vi "Read VI Refnum.vi"(8 "error in (no error)":errorcluster, 11 "Bioreactor in":refnum<class "Bioreactor.lvclass">) -> (0 "error out":errorcluster, 2 "VI Refnum":refnum<vi>, 3 "Bioreactor out":refnum<class "Bioreactor.lvclass">)   [LabVIEW 2012, in "Bioreactor Actor.lvlib" / "Bioreactor.lvclass"]
uses:
  Bioreactor.lvclass
  Bioreactor.lvclass/Bioreactor.ctl
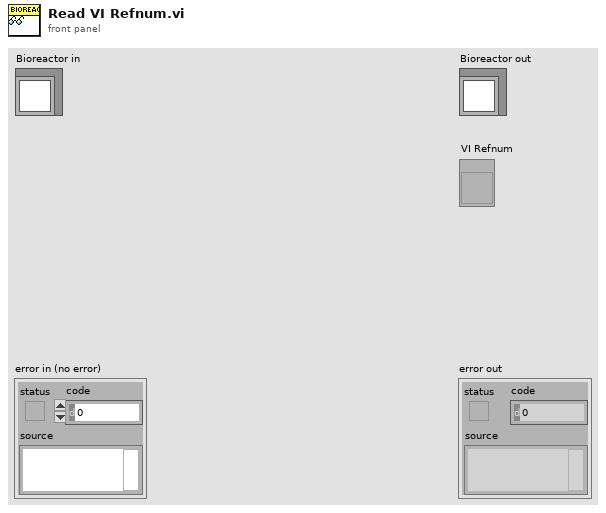
[diagram p1: front panel]
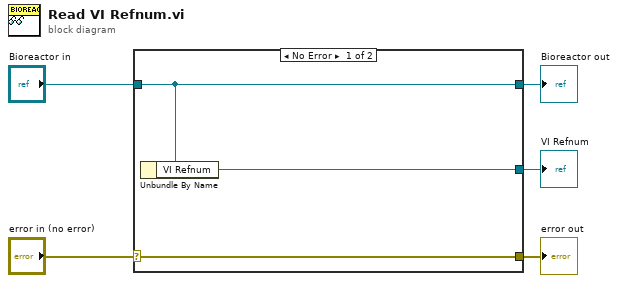
[diagram p0: block diagram]
diagram:
  n1 = case shown="No Error" "error in (no error)" {
    selector: "error in (no error)" -> [w8 w9]
    tunnel: [w8 w9] -> w4
    tunnel: [w7 w10] -> w2
    tunnel: "Bioreactor in" -> [w7 w10]
    tunnel: [w6 _] -> w1
    frame No Error {
      n2 = Unbundle By Name(w7) -> ("VI Refnum"=w6:refnum<vi>)
    }
    frame Error {
    }
  }
  "error out" <- w4
  "Bioreactor out" <- w2
  "VI Refnum" <- w1
